vi "SP Format Ch Data Plot.vi"(6 "Channel":i8=1, 7 "Marker Values Ref":refnum<vi>, 8 "error in (no error)":errorcluster, 9 "CH Controls":T1={"Trace On"=TRUE, "Measure"=0, "Format"=0, "Autoscale"=TRUE, "Reference"=0.0, "\nRefUnit"="dB/Div", "Position"=5.0, "Scale"=10.0, "ScaleUnit"="dB/Div", "LimitOn"=TRUE, "LimitFill"=FALSE, "Display Data"=0, "Show Markers"=TRUE, "SXX"=""} {"Reference" format="%#.2g"; "Display Data" items=["Data", "Memory", "Data/Memory"]; "Format" items=["Log Mag", "Phase", "Expanded Phase", "Delay", "Smith", "Polar", "Lin Mag", "SWR", "Loss", "Real", "Imaginary"]; "Scale" min=0.001 step=1.0 format="%#.2g"; "Position" min=0.0 max=10.0}, 10 "CH Control":refnum<vi>, 11 "Plot Reference":refnum<vi>) -> (0 "error out":errorcluster, 1 "dup CH Controls":T1={"Trace On"=TRUE, "Measure"=0, "Format"=0, "Autoscale"=TRUE, "Reference"=0.0, "\nRefUnit"="dB/Div", "Position"=5.0, "Scale"=10.0, "ScaleUnit"="dB/Div", "LimitOn"=TRUE, "LimitFill"=FALSE, "Display Data"=0, "Show Markers"=TRUE, "SXX"=""} {"Reference" format="%#.2g"; "Display Data" items=["Data", "Memory", "Data/Memory"]; "Format" items=["Log Mag", "Phase", "Expanded Phase", "Delay", "Smith", "Polar", "Lin Mag", "SWR", "Loss", "Real", "Imaginary"]; "Scale" min=0.001 step=1.0 format="%#.2g"; "Position" min=0.0 max=10.0})   [LabVIEW 2011]
uses:
  TypeDefs/SP Display Trace Controls.ctl
  TypeDefs/SP Display Format.ctl
  TypeDefs/SP Display Data.ctl
  TypeDefs/SP Plot Cluster Object.ctl
panel:
  # "Div"
  # "Div"
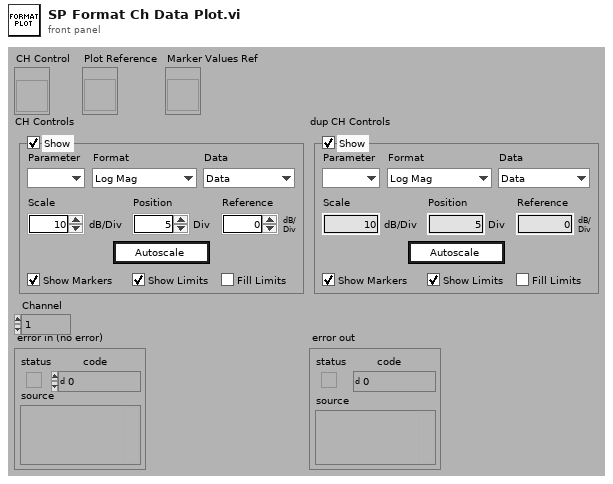
[diagram p1: front panel]
types:
  T1 = typedef "SP Display Trace Controls.ctl" = cluster{"Trace On":bool, "Measure":i32, "Format":T2, "Autoscale":bool, "Reference":dbl, "\nRefUnit":string, "Position":dbl, "Scale":dbl, "ScaleUnit":string, "LimitOn":bool, "LimitFill":bool, "Display Data":T3, "Show Markers":bool, "SXX":string}
  T2 = typedef "SP Display Format.ctl" = i32
  T3 = typedef "SP Display Data.ctl" = u16
  T4 = typedef "SP Plot Cluster Object.ctl" = enum16{"Plot", "CH Reference", "CH Label", "Start Label", "Stop Label", "Units Label", "Selected?", "CH Markers"}
  T5 = enum8{"Enabled", "Disabled", "Disabled and Grayed Out"}
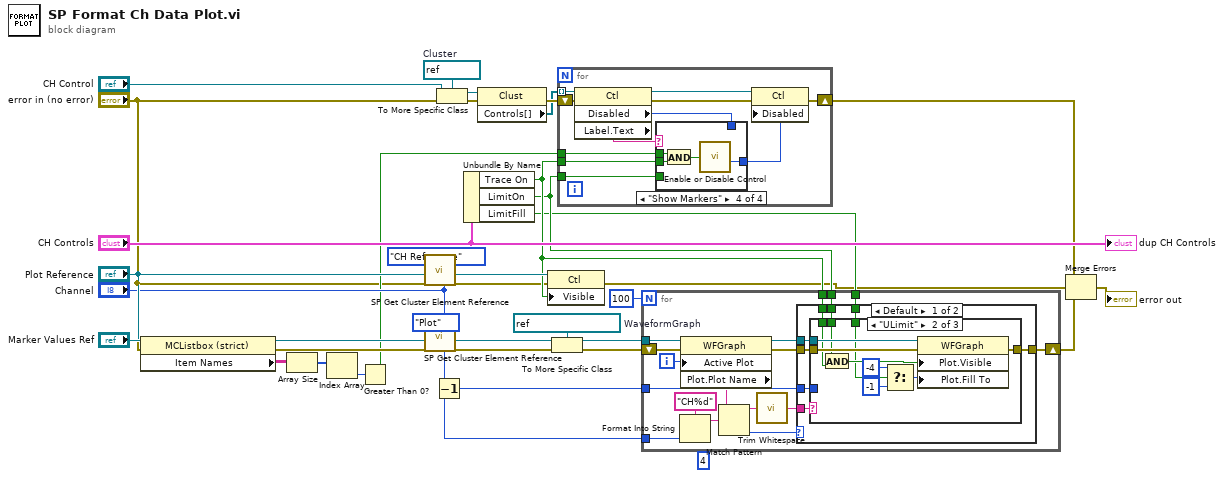
[diagram p0: block diagram]
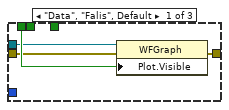
[diagram p2: hidden frame]
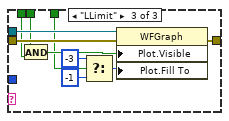
[diagram p3: hidden frame]
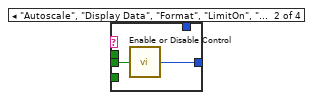
[diagram p6: hidden frame]
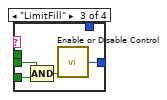
[diagram p7: hidden frame]
diagram:
  (unwired) 4
  w20 = refnum<vi> refnum  # WaveformGraph
  w32 = refnum<vi> refnum  # Cluster
  n1 = property class="MCListbox (strict)"(reference="Marker Values Ref", error in="error in (no error)") -> (error out=w8:errorcluster, "Item Names"=w13:string[][])  [unwired: 1 out]
  n2 = Array Size(array=w13) -> (size(s)=w12:i32[])
  n3 = Index Array(array=w12) -> (element=w11:i32)  [unwired: 1 in]
  n4 = Greater Than 0?(x=w11) -> (x > 0?=w7:bool)
  n5 = call "SP Get Cluster Element Reference.vi"("Channel"="Channel", "Element"=SP_Plot_Cluster_Object."CH Reference", "Plot Reference"="Plot Reference") -> ("Element Reference"=w24:refnum<vi>)  [unwired: 6 out]
  n6 = call "SP Get Cluster Element Reference.vi"("Channel"="Channel", "Element"=SP_Plot_Cluster_Object."Plot", "Plot Reference"="Plot Reference") -> ("Element Reference"=w19:refnum<vi>)  [unwired: 6 out]
  n7 = Decrement(x="Channel") -> (x-1=w4:i8)
  n8 = To More Specific Class(target class=w32, reference="CH Control", error in="error in (no error)") -> (specific class reference=w31:refnum<vi>, error out=w30:errorcluster)
  n9 = Unbundle By Name("CH Controls") -> ("Trace On"=w17:bool, "LimitOn"=w16:bool, "LimitFill"=w15:bool)
  n10 = property class="Clust"(reference=w31, error in=w30) -> (error out=w28:errorcluster, "Controls[]"=w27:refnum<vi>[])  [unwired: 1 out]
  n11 = property class="Ctl"(reference=w24, error in="error in (no error)", "Visible"=w17) -> (error out=w2:errorcluster)  [unwired: 1 out]
  n12 = To More Specific Class(target class=w20, reference=w19, error in=w8) -> (specific class reference=w5:refnum<vi>, error out=w18:errorcluster)
  n13 = for {
    shift-right: [w39] -> w1
    shift-left: w28 -> [w42]
    tunnel: w27 -> [w43] mode=indexing
    tunnel: w17 -> [w41]
    tunnel: w16 -> [w40]
    tunnel: w7 -> [w33]
    n14 = property class="Ctl"(reference=w43, error in=w42) -> (reference out=w38:refnum<vi>, error out=w36:errorcluster, "Disabled"=w34:u8, "Label.Text"=w35:string)
    n15 = case shown="\"Show Markers\"" w35 {
      tunnel: w41 -> [_ w46 w50 w53]
      tunnel: w40 -> [_ _ w49 _]
      tunnel: [w44 w45 w47 w54] -> w37
      tunnel: w34 -> [w44 _ _ _]
      tunnel: w33 -> [_ _ _ w51]
      frame Default {
      }
      frame "Autoscale", "Display Data", "Format", "LimitOn", "Measure", "Position", "Reference", "Scale" {
        n16 = call "Enable or Disable Control.vi"("Enable? (T)"=w46) -> ("Enable\\Disable"=w45:T5)
      }
      frame "LimitFill" {
        n17 = Compound Arithmetic op=AND(w50, w49) -> (w48:bool)
        n18 = call "Enable or Disable Control.vi"("Enable? (T)"=w48) -> ("Enable\\Disable"=w47:T5)
      }
      frame "Show Markers" {
        n19 = And(x=w51, y=w53) -> (x .and. y?=w52:bool)
        n20 = call "Enable or Disable Control.vi"("Enable? (T)"=w52) -> ("Enable\\Disable"=w54:T5)
      }
    }
    n21 = property class="Ctl"(reference=w38, error in=w36, "Disabled"=w37) -> (error out=w39:errorcluster)  [unwired: 1 out]
  }
  n22 = for {
    N: 100 -> [_]
    tunnel: w5 -> [w61]
    shift-right: [w70] -> w3
    shift-left: w18 -> [w62]
    tunnel: w4 -> [w71]
    tunnel: w17 -> [w69]
    tunnel: "Channel" -> [w64]
    tunnel: w16 -> [w56]
    tunnel: w15 -> [w55]
    i -> [w68]
    n23 = Format Into String(format string="CH%d", w64) -> (resulting string=w65:string)  [unwired: 2 in, 1 out]
    n24 = property class="WFGraph"(reference=w61, error in=w62, "Active Plot"=w68) -> (reference out=w60:refnum<vi>, error out=w59:errorcluster, "Plot.Plot Name"=w67:string)
    n25 = Match Pattern(string=w67, regular expression=w65) -> (before substring=w58:string, offset past match=w63:i32)  [unwired: 3 out]
    n26 = call <vilib>:"Trim Whitespace.vi"("string"=w58) -> ("trimmed string"=w57:string)  [unwired: 1 in]
    n27 = case shown="Default" w63 {
      tunnel: w60 -> [w79 _]
      tunnel: w59 -> [w78 w104]
      tunnel: w71 -> [w77 _]
      tunnel: [w76 w104] -> w70
      tunnel: w69 -> [w75 _]
      tunnel: w57 -> [w74 _]
      tunnel: w56 -> [w73 _]
      tunnel: w55 -> [w72 _]
      frame Default {
        n28 = case shown="\"ULimit\"" w74 {
          tunnel: w79 -> [w80 w91 w101]
          tunnel: w78 -> [w81 w92 w102]
          tunnel: w77 -> [_ _ _]
          tunnel: [w83 w93 w103] -> w76
          tunnel: w75 -> [w82 w90 w100]
          tunnel: w73 -> [_ w88 w98]
          tunnel: w72 -> [_ w84 w94]
          frame "Data", "Falis", Default {
            n29 = property class="WFGraph"(reference=w80, error in=w81, "Plot.Visible"=w82) -> (error out=w83:errorcluster)  [unwired: 1 out]
          }
          frame "ULimit" {
            n30 = And(x=w88, y=w90) -> (x .and. y?=w89:bool)
            n31 = Select(t=-4, s=w84, f=-1) -> (s? t:f=w87:i32)
            n32 = property class="WFGraph"(reference=w91, error in=w92, "Plot.Visible"=w89, "Plot.Fill To"=w87) -> (error out=w93:errorcluster)  [unwired: 1 out]
          }
          frame "LLimit" {
            n33 = And(x=w98, y=w100) -> (x .and. y?=w99:bool)
            n34 = Select(t=-3, s=w94, f=-1) -> (s? t:f=w97:i32)
            n35 = property class="WFGraph"(reference=w101, error in=w102, "Plot.Visible"=w99, "Plot.Fill To"=w97) -> (error out=w103:errorcluster)  [unwired: 1 out]
          }
        }
      }
      frame -1 {
      }
    }
  }
  n36 = Merge Errors(w1, w2, w3) -> (→"error out":errorcluster)
  "dup CH Controls" <- "CH Controls"
